vi "Controller Initialize Configuration.vi"(8 "error in (no error)":errorcluster, 11 "FOFB Configuration":T1) -> (0 "error out":errorcluster, 3 "FOFB Configuration":T1)   [LabVIEW 2011, in "Controller VIs.lvlib"]
uses:
  Controller VIs.lvlib
  Types Definitions/Type FOFB Configuration.ctl
  Types Definitions/Type FOFB Parameters.ctl
  Types Definitions/Type Network Configuration.ctl
  Types Definitions/Type FA Configuration.ctl
  Types Definitions/Type Response Matrix Measurement Configuration.ctl
  Types Definitions/Type Correction Algorithm Configuration.ctl
  Types Definitions/Type Acquisition Network Configuration.ctl
  Types Definitions/Type Actuation Network Configuration.ctl
  Types Definitions/Type PID Parameters.ctl
  Types Definitions/Type Operation Mode State.ctl
  Types Definitions/Type Control FOFB Configuration Out.ctl
  Types Definitions/Type Control FOFB Configuration In.ctl
  Controller Global Variables/LNLS Control FOFB Configuration Out.vi
  Controller Global Variables/LNLS Control FOFB Configuration In.vi
  Type Definitions.lvlib
  Controller Global Variables.lvlib
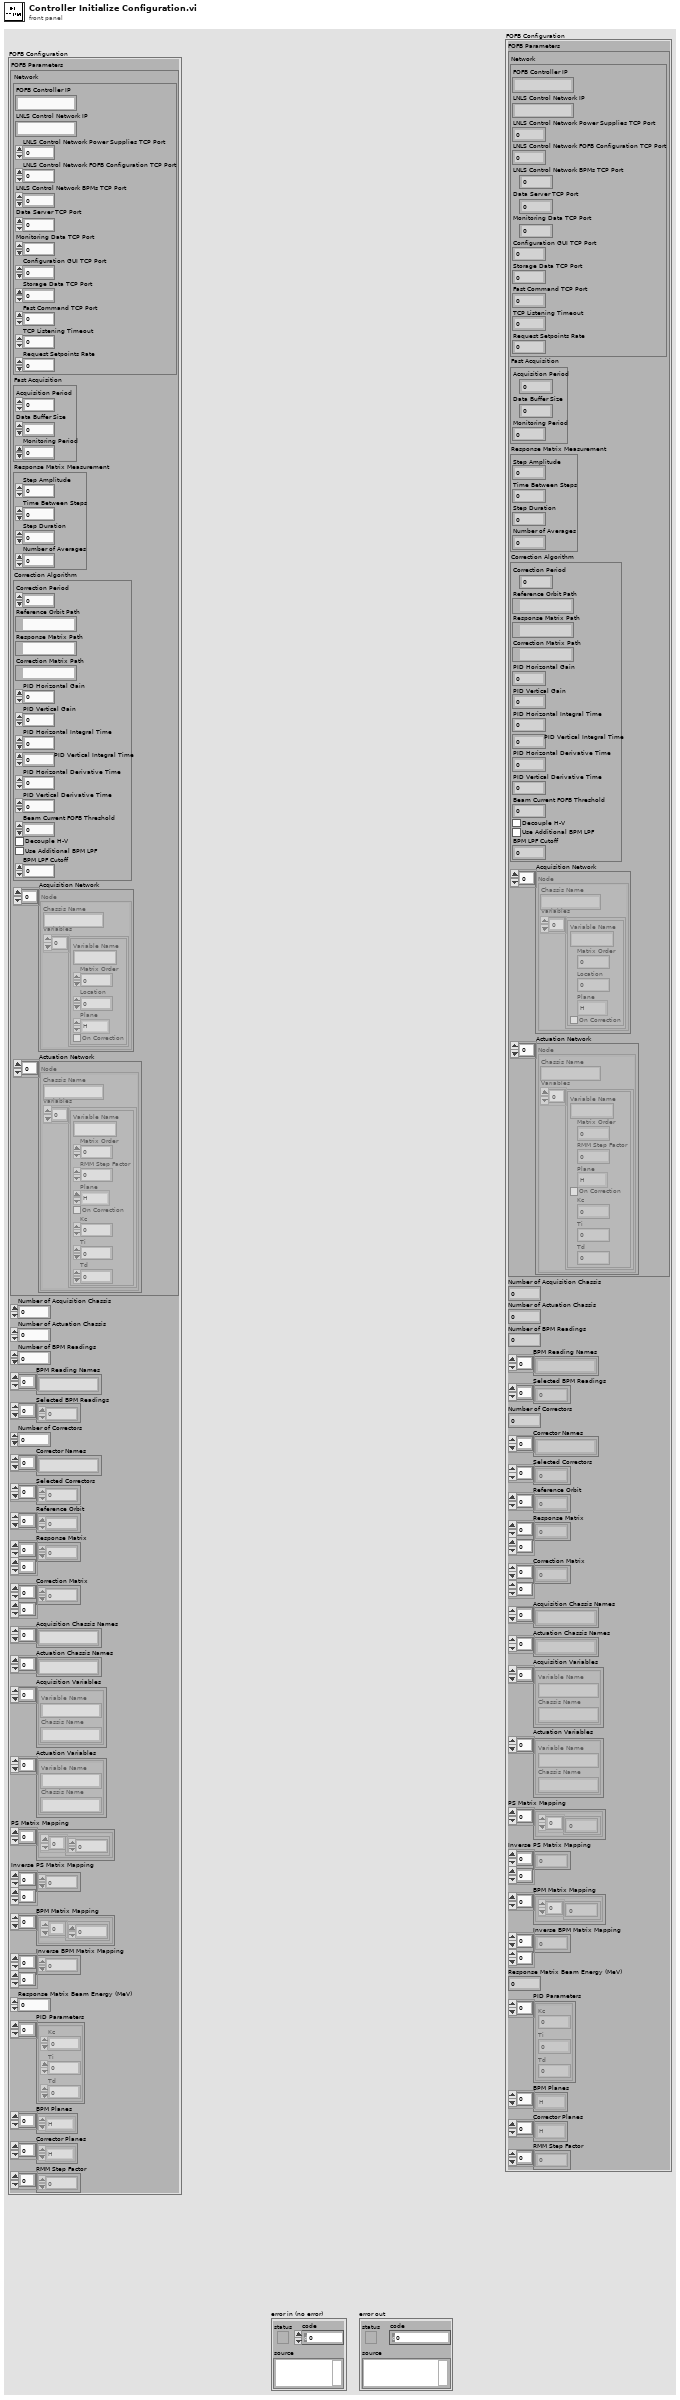
[diagram p1: front panel]
types:
  T1 = typedef "Type Definitions.lvlib/Type FOFB Configuration.ctl" = cluster{"FOFB Parameters":T2, "Number of Acquisition Chassis":i32, "Number of Actuation Chassis":i32, "Number of BPM Readings":i32, "BPM Reading Names":string[], "Selected BPM Readings":u32[], "Number of Correctors":i32, "Corrector Names":string[], "Selected Correctors":u32[], "Reference Orbit":dbl[], "Response Matrix":dbl[][], "Correction Matrix":dbl[][], "Acquisition Chassis Names":string[], "Actuation Chassis Names":string[], "Acquisition Variables":cluster{"Variable Name":string, "Chassis Name":string}[], "Actuation Variables":cluster{"Variable Name":string, "Chassis Name":string}[], "PS Matrix Mapping":cluster{u32[]}[], "Inverse PS Matrix Mapping":u32[][], "BPM Matrix Mapping":cluster{u32[]}[], "Inverse BPM Matrix Mapping":u32[][], "Response Matrix Beam Energy (MeV)":dbl, "PID Parameters":T9[], "BPM Planes":enum8{"H", "V"}[], "Corrector Planes":enum8{"H", "V"}[], "RMM Step Factor":dbl[]}
  T2 = typedef "Type Definitions.lvlib/Type FOFB Parameters.ctl" = cluster{"Network":T3, "Fast Acquisition":T4, "Response Matrix Measurement":T5, "Correction Algorithm":T6, "Acquisition Network":T7, "Actuation Network":T8}
  T3 = typedef "Type Definitions.lvlib/Type Network Configuration.ctl" = cluster{"FOFB Controller IP":string, "LNLS Control Network IP":string, "LNLS Control Network Power Supplies TCP Port":u16, "LNLS Control Network FOFB Configuration TCP Port":u16, "LNLS Control Network BPMs TCP Port":u16, "Data Server TCP Port":u16, "Monitoring Data TCP Port":u16, "Configuration GUI TCP Port":u16, "Storage Data TCP Port":u16, "Fast Command TCP Port":u16, "TCP Listening Timeout":i32, "Request Setpoints Rate":u16}
  T4 = typedef "Type Definitions.lvlib/Type FA Configuration.ctl" = cluster{"Acquisition Period":u32, "Data Buffer Size":u32, "Monitoring Period":u32}
  T5 = typedef "Type Definitions.lvlib/Type Response Matrix Measurement Configuration.ctl" = cluster{"Step Amplitude":dbl, "Time Between Steps":u32, "Step Duration":u32, "Number of Averages":u32}
  T6 = typedef "Type Definitions.lvlib/Type Correction Algorithm Configuration.ctl" = cluster{"Correction Period":u32, "Reference Orbit Path":path, "Response Matrix Path":path, "Correction Matrix Path":path, "PID Horizontal Gain":dbl, "PID Vertical Gain":dbl, "PID Horizontal Integral Time":dbl, "PID Vertical Integral Time":dbl, "PID Horizontal Derivative Time":dbl, "PID Vertical Derivative Time":dbl, "Beam Current FOFB Threshold":dbl, "Decouple H-V":bool, "Use Additional BPM LPF":bool, "BPM LPF Cutoff":dbl}
  T7 = typedef "Type Definitions.lvlib/Type Acquisition Network Configuration.ctl" = cluster{"Chassis Name":string, "Variables":cluster{"Variable Name":string, "Matrix Order":u32, "Location":dbl, "Plane":enum8{"H", "V"}, "On Correction":bool}[]}[]
  T8 = typedef "Type Definitions.lvlib/Type Actuation Network Configuration.ctl" = cluster{"Chassis Name":string, "Variables":cluster{"Variable Name":string, "Matrix Order":u32, "RMM Step Factor":dbl, "Plane":enum8{"H", "V"}, "On Correction":bool, "Kc":dbl, "Ti":dbl, "Td":dbl}[]}[]
  T9 = typedef "Type Definitions.lvlib/Type PID Parameters.ctl" = cluster{"Kc":fxp<+/-,16,8>, "Ti":fxp<+/-,16,8>, "Td":fxp<+/-,16,8>}
  T10 = typedef "Type Definitions.lvlib/Type Control FOFB Configuration In.ctl" = cluster{"Status":u16, "Operation Mode":T11, "PID Horizontal Gain":sgl, "PID Vertical Gain":sgl, "PID Horizontal Integral Time":sgl, "PID Vertical Integral Time":sgl, "PID Horizontal Derivative Time":sgl, "PID Vertical Derivative Time":sgl, "Fast Command Enabled":bool}
  T11 = typedef "Type Definitions.lvlib/Type Operation Mode State.ctl" = enum8{"Idle Mode", "Manual Mode", "FOFB Mode", "RMM Mode"}
  T12 = typedef "Type Definitions.lvlib/Type Control FOFB Configuration Out.ctl" = cluster{"Status":u16, "Operation Mode":T11, "PID Horizontal Gain":sgl, "PID Vertical Gain":sgl, "PID Horizontal Integral Time":sgl, "PID Vertical Integral Time":sgl, "PID Horizontal Derivative Time":sgl, "PID Vertical Derivative Time":sgl, "Fast Command Enabled":bool, "RMS Horizontal Distortion":dbl, "RMS Vertical Distortion":dbl, "Timestamp":dbl}
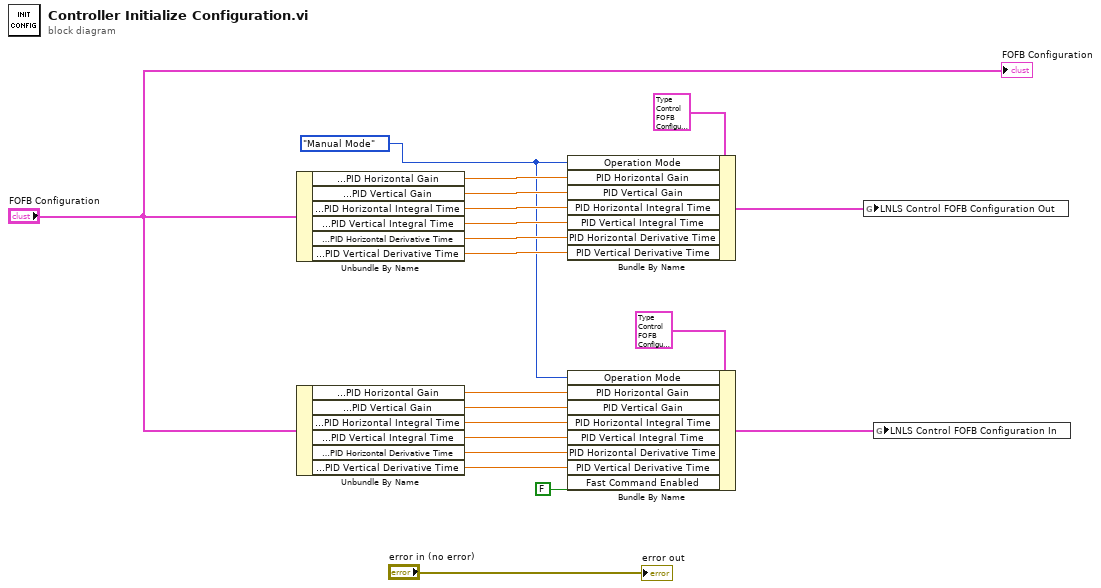
[diagram p0: block diagram]
diagram:
  w2 = Type_Operation_Mode_State."Manual Mode" ("Operation Mode")
  n1 = Unbundle By Name("FOFB Configuration") -> ("FOFB Parameters.Correction Algorithm.PID Horizontal Gain"=w15:dbl, "FOFB Parameters.Correction Algorithm.PID Vertical Gain"=w16:dbl, "FOFB Parameters.Correction Algorithm.PID Horizontal Integral Time"=w17:dbl, "FOFB Parameters.Correction Algorithm.PID Vertical Integral Time"=w18:dbl, "FOFB Parameters.Correction Algorithm.PID Horizontal Derivative Time"=w19:dbl, "FOFB Parameters.Correction Algorithm.PID Vertical Derivative Time"=w20:dbl)
  n2 = Unbundle By Name("FOFB Configuration") -> ("FOFB Parameters.Correction Algorithm.PID Horizontal Gain"=w11:dbl, "FOFB Parameters.Correction Algorithm.PID Vertical Gain"=w10:dbl, "FOFB Parameters.Correction Algorithm.PID Horizontal Integral Time"=w9:dbl, "FOFB Parameters.Correction Algorithm.PID Vertical Integral Time"=w8:dbl, "FOFB Parameters.Correction Algorithm.PID Horizontal Derivative Time"=w7:dbl, "FOFB Parameters.Correction Algorithm.PID Vertical Derivative Time"=w6:dbl)
  n3 = Bundle By Name(cluster=T12 {"Status"=0, "Operation Mode"=enum."Manual Mode", "PID Horizontal Gain"=0.0, "PID Vertical Gain"=0.0, "PID Horizontal Integral Time"=0.0, "PID Vertical Integral Time"=0.0, "PID Horizontal Derivative Time"=0.0, "PID Vertical Derivative Time"=0.0, "Fast Command Enabled"=FALSE, "RMS Horizontal Distortion"=0.0, "RMS Vertical Distortion"=0.0, "Timestamp"=0.0} ("LNLS Control FOFB Configuration Out"), "Operation Mode"=w2, "PID Horizontal Gain"=w15, "PID Vertical Gain"=w16, "PID Horizontal Integral Time"=w17, "PID Vertical Integral Time"=w18, "PID Horizontal Derivative Time"=w19, "PID Vertical Derivative Time"=w20) -> (w12:T12)
  n4 = Bundle By Name(cluster=T10 {"Status"=0, "Operation Mode"=enum."Idle Mode", "PID Horizontal Gain"=0.0, "PID Vertical Gain"=0.0, "PID Horizontal Integral Time"=0.0, "PID Vertical Integral Time"=0.0, "PID Horizontal Derivative Time"=0.0, "PID Vertical Derivative Time"=0.0, "Fast Command Enabled"=FALSE} ("LNLS Control FOFB Configuration In"), "Operation Mode"=w2, "PID Horizontal Gain"=w11, "PID Vertical Gain"=w10, "PID Horizontal Integral Time"=w9, "PID Vertical Integral Time"=w8, "PID Horizontal Derivative Time"=w7, "PID Vertical Derivative Time"=w6, "Fast Command Enabled"=FALSE) -> (w3:T10)
  n5 = global write "LNLS Control FOFB Configuration Out.vi" "LNLS Control FOFB Configuration Out"(w12) -> ()
  n6 = global write "LNLS Control FOFB Configuration In.vi" "LNLS Control FOFB Configuration In"(w3) -> ()
  "FOFB Configuration" <- "FOFB Configuration"
  "error out" <- "error in (no error)"
